vi "RT fast measure v2.vi"(8 "error in":errorcluster, 11 "FPGA DAQ1":refnum<k20>) -> (0 "error out":errorcluster)   [LabVIEW 2024]
uses:
  RT fast data.ctl
  <vilib>/LabVIEW Targets/FPGA/cRIO/shared/nicrio_ModuleControls/nicrio_cRIO-9775_RecordDataRates4ChansRing.ctl
  <vilib>/LabVIEW Targets/FPGA/cRIO/shared/nicrio_ModuleControls/nicrio_BasicConversionTime.ctl
  Ramps.ctl
  <vilib>/FPGAPlugInAG/Dynamic/niLvFpga_Reset_Dynamic.vi
  <vilib>/Utility/error.llb/Error Cluster From Error Code.vi
  <vilib>/rvi/errors/niLvFpgaAdjustHostInterfaceError.vi
  <vilib>/FPGAPlugInAG/Dynamic/niLvFpga_Run_Dynamic.vi
  <vilib>/RVI Host/nirviSupport.llb/nirviErrorClusterFromErrorCode.vi
  <vilib>/rvi/interface/nirviMethod/nirviMethod.xnode
  <vilib>/rvi/interface/nirviReadWriteControl/nirviReadWriteControl.xnode
  <resource>/objmgr/ni.dex.rc
  <vilib>/rvi/interface/nirviMethod/StockFPGA_InlinedMethodWaitForSingleIRQ.vi
  <vilib>/FPGAPlugInAG/Dynamic/niLvFpga_WaitOnIrq_Dynamic.vi
  <vilib>/FPGAPlugInAG/Dynamic/niLvFpga_AcknowledgeIrq_Dynamic.vi
  <vilib>/FPGAPlugInAG/Dynamic/niLvFpga_ReadFifo_Dynamic.vi
  <vilib>/rvi/errors/niLvFpgaMergeErrorWithErrorCode.vi
  NiFpgaLv.dll
  <vilib>/rvi/interface/Simulation/niFpgaSimulationCallBeginRW.vi
panel:
  in  "Parameters":T1={"Records Num"=10000, "AI Trigger Configuration"={"Trigger Slope"=enum."Positive", "Trigger Level"=0.1298828125, "Hystesis Value"=0.0, "AI Channel"=0}, "Record PreTrigger Samples"=1, "Record Samples"=16, "Ic Cut off or curve"=TRUE, "Record Data Rate"=1, "Wait before trigger us"=10100, "Cutoff delay usec"=0, "Timing Mode"=enum."High Resolution", "Trigger length ticks"=15000, "Timeout"=-1, "Ramps"={"Amp"=0.0, "Delay time 10us"=1, "Ramp1 time 10us"=1000, "Ramp2 time 10us"=2000, "Ramp3 time 10us"=1000, "End time 10us"=1}} {"Record Data Rate" items=["20.000 MS/s (NI 9775)"=1, "10.00 MS/s (NI 9775)"=2, "6.667 MS/s (NI 9775)"=3, "5.000 MS/s (NI 9775)"=4, "2.500 MS/s (NI 9775)"=8, "1.667 MS/s (NI 9775)"=12, "1.250 MS/s (NI 9775)"=16, "1.000 MS/s (NI 9775)"=20, "833.333 KS/s (NI 9775)"=24, "714.286 KS/s (NI 9775)"=28, "625.000 KS/s (NI 9775)"=32, "555.556 KS/s (NI 9775)"=36, "500.000 KS/s (NI 9775)"=40, "454.545 KS/s (NI 9775)"=44, "416.667 KS/s (NI 9775)"=48, "384.615 KS/s (NI 9775)"=52, "357.143 KS/s (NI 9775)"=56, "333.333 KS/s (NI 9775)"=60, "312.500 KS/s (NI 9775)"=64, "294.118 KS/s (NI 9775)"=68, "277.778 KS/s (NI 9775)"=72, "263.158 KS/s (NI 9775)"=76, "250.000 KS/s (NI 9775)"=80, "238.095 KS/s (NI 9775)"=84, "227.273 KS/s (NI 9775)"=88, "217.391 KS/s (NI 9775)"=92, "208.333 KS/s (NI 9775)"=96, "200.000 KS/s (NI 9775)"=100, "192.308 KS/s (NI 9775)"=104, "185.185 KS/s (NI 9775)"=108, "178.571 KS/s (NI 9775)"=112, "172.414 KS/s (NI 9775)"=116, "166.667 KS/s (NI 9775)"=120, "161.290 KS/s (NI 9775)"=124, "156.250 KS/s (NI 9775)"=128, "151.515 KS/s (NI 9775)"=132, "147.059 KS/s (NI 9775)"=136, "142.857 KS/s (NI 9775)"=140, "138.889 KS/s (NI 9775)"=144, "135.135 KS/s (NI 9775)"=148, "131.579 KS/s (NI 9775)"=152, "128.205 KS/s (NI 9775)"=156, "125.000 KS/s (NI 9775)"=160, "121.951 KS/s (NI 9775)"=164, "119.048 KS/s (NI 9775)"=168, "116.279 KS/s (NI 9775)"=172, "113.636 KS/s (NI 9775)"=176, "111.111 KS/s (NI 9775)"=180, "108.696 KS/s (NI 9775)"=184, "106.383 KS/s (NI 9775)"=188, "104.167 KS/s (NI 9775)"=192, "102.041 KS/s (NI 9775)"=196, "100.000 KS/s (NI 9775)"=200, "50.000 KS/s (NI 9775)"=400, "33.333 KS/s (NI 9775)"=600, "25.000 KS/s (NI 9775)"=800, "20.000 KS/s (NI 9775)"=1000, "16.667 KS/s (NI 9775)"=1200, "14.286 KS/s (NI 9775)"=1400, "12.500 KS/s (NI 9775)"=1600, "11.111 KS/s (NI 9775)"=1800, "10.000 KS/s (NI 9775)"=2000, "9.091 KS/s (NI 9775)"=2200, "8.333 KS/s (NI 9775)"=2400, "7.692 KS/s (NI 9775)"=2600, "7.143 KS/s (NI 9775)"=2800, "6.667 KS/s (NI 9775)"=3000, "6.250 KS/s (NI 9775)"=3200, "5.882 KS/s (NI 9775)"=3400, "5.556 KS/s (NI 9775)"=3600, "5.000 KS/s (NI 9775)"=4000, "4.762 KS/s (NI 9775)"=4200, "4.545 KS/s (NI 9775)"=4400, "4.348 KS/s (NI 9775)"=4600, "4.167 KS/s (NI 9775)"=4800, "4.000 KS/s (NI 9775)"=5000, "3.846 KS/s (NI 9775)"=5200, "3.571 KS/s (NI 9775)"=5600, "3.333 KS/s (NI 9775)"=6000, "3.125 KS/s (NI 9775)"=6400, "2.941 KS/s (NI 9775)"=6800, "2.778 KS/s (NI 9775)"=7200, "2.632 KS/s (NI 9775)"=7600, "2.500 KS/s (NI 9775)"=8000, "2.381 KS/s (NI 9775)"=8400, "2.273 KS/s (NI 9775)"=8800, "2.174 KS/s (NI 9775)"=9200, "2.083 KS/s (NI 9775)"=9600, "2.000 KS/s (NI 9775)"=10000, "1.923 KS/s (NI 9775)"=10400, "1.852 KS/s (NI 9775)"=10800, "1.786 KS/s (NI 9775)"=11200, "1.724 KS/s (NI 9775)"=11600, "1.667 KS/s (NI 9775)"=12000, "1.613 KS/s (NI 9775)"=12400, "1.563 KS/s (NI 9775)"=12800, "1.515 KS/s (NI 9775)"=13200, "1.471 KS/s (NI 9775)"=13600, "1.429 KS/s (NI 9775)"=14000, "1.389 KS/s (NI 9775)"=14400, "1.351 KS/s (NI 9775)"=14800, "1.316 KS/s (NI 9775)"=15200, "1.282 KS/s (NI 9775)"=15600, "1.250 KS/s (NI 9775)"=16000, "1.220 KS/s (NI 9775)"=16400, "1.190 KS/s (NI 9775)"=16800, "1.163 KS/s (NI 9775)"=17200, "1.136 KS/s (NI 9775)"=17600, "1.111 KS/s (NI 9775)"=18000, "1.087 KS/s (NI 9775)"=18400, "1.064 KS/s (NI 9775)"=18800, "1.042 KS/s (NI 9775)"=19200, "1.020 KS/s (NI 9775)"=19600, "1.000 KS/s (NI 9775)"=20000, "0.980 KS/s (NI 9775)"=20400, "0.962 KS/s (NI 9775)"=20800, "0.943 KS/s (NI 9775)"=21200, "0.926 KS/s (NI 9775)"=21600, "0.909 KS/s (NI 9775)"=22000, "0.893 KS/s (NI 9775)"=22400, "0.877 KS/s (NI 9775)"=22800, "0.862 KS/s (NI 9775)"=23200, "0.847 KS/s (NI 9775)"=23600, "0.833 KS/s (NI 9775)"=24000, "0.820 KS/s (NI 9775)"=24400, "0.806 KS/s (NI 9775)"=24800, "0.794 KS/s (NI 9775)"=25200, "0.781 KS/s (NI 9775)"=25600, "0.694 KS/s (NI 9775)"=28800, "0.625 KS/s (NI 9775)"=32000, "0.568 KS/s (NI 9775)"=35200, "0.521 KS/s (NI 9775)"=38400, "0.446 KS/s (NI 9775)"=44800, "0.391 KS/s (NI 9775)"=51200, "0.347 KS/s (NI 9775)"=57600, "0.313 KS/s (NI 9775)"=64000]}
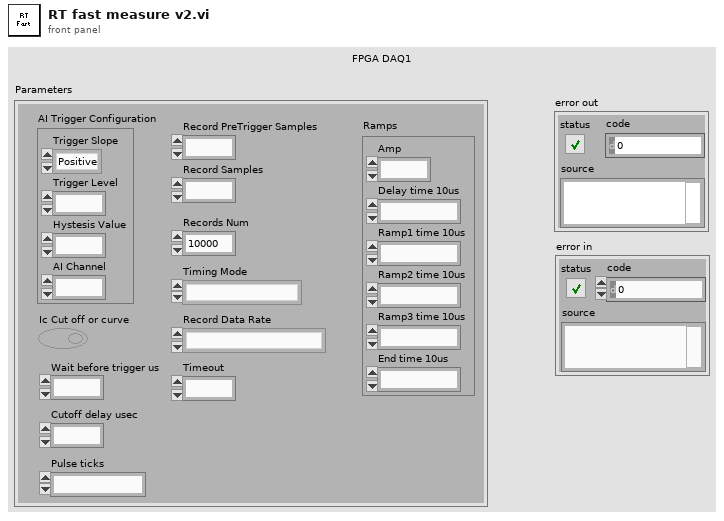
[diagram p1: front panel]
types:
  T1 = typedef "RT fast data.ctl" = cluster{"Records Num":i32, "AI Trigger Configuration":cluster{"Trigger Slope":enum8{"Positive", "Negative"}, "Trigger Level":fxp<+/-,17,5>, "Hystesis Value":fxp<+,16,4>, "AI Channel":u8}, "Record PreTrigger Samples":u32, "Record Samples":u32, "Ic Cut off or curve":bool, "Record Data Rate":T2, "Wait before trigger us":u32, "Cutoff delay usec":u32, "Timing Mode":T3, "Trigger length ticks":u32, "Timeout":i32, "Ramps":T4}
  T2 = typedef "nicrio_cRIO-9775_RecordDataRates4ChansRing.ctl" = u16
  T3 = typedef "nicrio_BasicConversionTime.ctl" = enum8{"High Speed", "High Resolution"}
  T4 = typedef "Ramps.ctl" = cluster{"Amp":fxp<+/-,20,5>, "Delay time 10us":i32, "Ramp1 time 10us":i32, "Ramp2 time 10us":i32, "Ramp3 time 10us":i32, "End time 10us":i32}
  T5 = cluster{"Trigger Slope":enum8{"Positive", "Negative"}, "Trigger Level":fxp<+/-,17,5>, "Hystesis Value":fxp<+,16,4>, "AI Channel":u8}
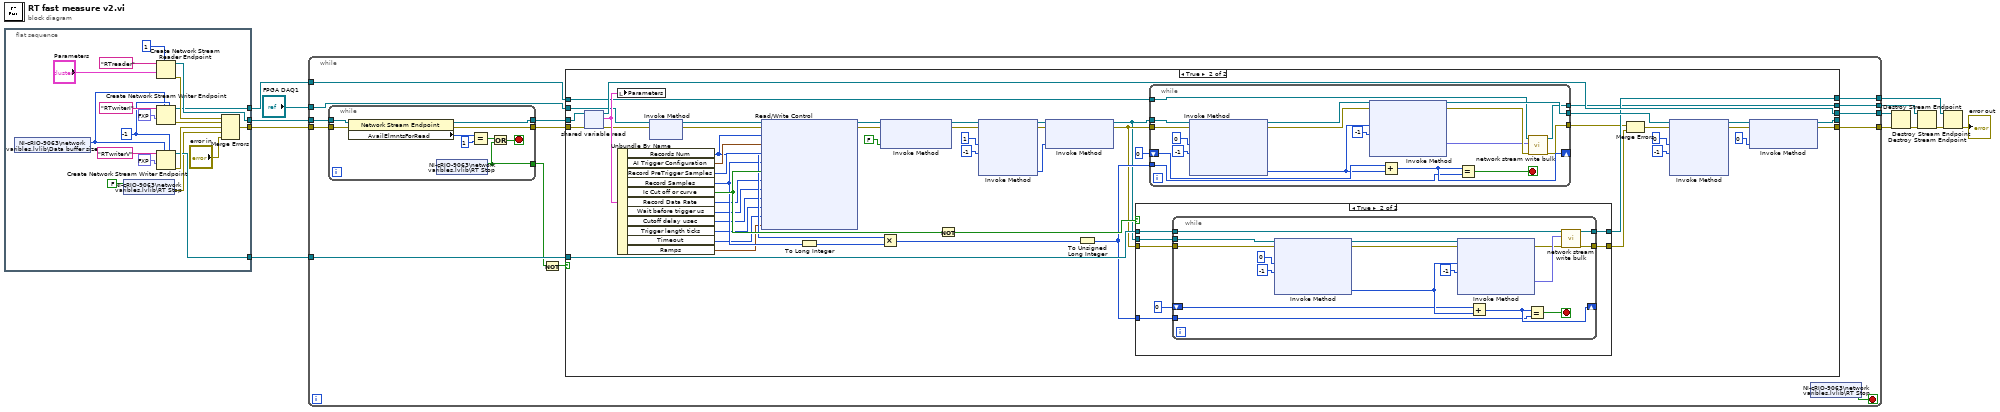
[diagram p0: block diagram]
diagram:
  n1 = flat-sequence {
    tunnel: [w29] -> w12
    tunnel: [w19] -> w11
    tunnel: [w18] -> w6
    tunnel: [w17] -> w5
    frame #0 {
      w24 = -1 ("timeout in ms (-1)")
      n2 = shared-variable "NI-cRIO-9063\\network varibles.lvlib\\Data buffer size"() -> (w23:i32)  [unwired: 1 in, 1 out]
      n3 = shared-variable "NI-cRIO-9063\\network varibles.lvlib\\RT Stop"(FALSE ("RT Stop")) -> (error out=w15:errorcluster)  [unwired: 1 in]
      n4 = Create Network Stream Reader Endpoint(7:1 ("reader buffer size"), 9:"Parameters", 11:"RTreader" ("reader name")) -> (0:w22:errorcluster, 3:w29:refnum<k21>)  [unwired: 4 in]
      n5 = Create Network Stream Writer Endpoint(5:w24, 7:w23, 9:fxp<+/-,17,5> 0.0, 11:"RTwriterI" ("writer name")) -> (0:w21:errorcluster, 3:w18:refnum<k21>)  [unwired: 3 in]
      n6 = Create Network Stream Writer Endpoint(5:w24, 7:w23, 9:fxp<+/-,17,5> 0.0, 11:"RTwriterV" ("writer name")) -> (0:w20:errorcluster, 3:w17:refnum<k21>)  [unwired: 3 in]
      n7 = Merge Errors(w22, w21, w20, w15, "error in") -> (w19:errorcluster)
    }
  }
  n8 = while {
    tunnel: w12 -> [w45]
    tunnel: w11 -> [w44]
    tunnel: [w34] -> w2
    tunnel: [w41] -> w10
    tunnel: w6 -> [w38]
    tunnel: w5 -> [w37]
    tunnel: [w36] -> w4
    tunnel: [w35] -> w3
    tunnel: "FPGA DAQ1" -> [w32]
    stop <- w40 stop-if-true
    n9 = while {
      tunnel: w45 -> [w154]
      tunnel: w44 -> [w153]
      tunnel: [w152] -> w43
      tunnel: [w151] -> w42
      tunnel: [w146] -> w33
      stop <- w147 stop-if-true
      n10 = property class="Network Stream Endpoint"(reference=w154, error in=w153) -> (reference out=w152:refnum<k21>, error out=w151:errorcluster, "AvailElmntsForRead"=w150:i32)
      n11 = shared-variable "NI-cRIO-9063\\network varibles.lvlib\\RT Stop"() -> (w146:bool)  [unwired: 1 in, 1 out]
      n12 = Equal?(x=w150, y=1) -> (x = y?=w148:bool)
      n13 = Or(x=w148, y=w146) -> (x .or. y?=w147:bool)
    }
    n14 = Not(x=w33) -> (.not. x?=w39:bool)
    n15 = case shown="True" w39 {
      tunnel: w43 -> [w49 w96]
      tunnel: w42 -> [w50 w65]
      tunnel: [w48 w88] -> _
      tunnel: [w50 w87] -> w34
      tunnel: [w49 w86] -> w41
      tunnel: w32 -> [w48 w66]
      tunnel: w38 -> [w47 w74]
      tunnel: w37 -> [w46 w76]
      tunnel: [w47 w73] -> w36
      tunnel: [w46 w75] -> w35
      frame False {
      }
      frame True {
        n16 = shared-variable-read(w96, w65) -> (w86:refnum<k21>, w64:errorcluster, w95:T1)  [unwired: 1 in, 1 out]
        n17 = local write "Parameters"(w95) -> ()
        n18 = Unbundle By Name(w95) -> ("Records Num"=w80:i32, "AI Trigger Configuration"=w98:T5, "Record PreTrigger Samples"=w97:u32, "Record Samples"=w79:u32, "Ic Cut off or curve"=w83:bool, "Record Data Rate"=w71:T2, "Wait before trigger us"=w67:u32, "Cutoff delay usec"=w63:u32, "Trigger length ticks"=w53:u32, "Timeout"=w52:i32, "Ramps"=w51:T4)
        n19 = xnode "Invoke Method"("FPGA VI Reference In"=w66, "error in"=w64) -> ("FPGA VI Reference Out"=w100:refnum<k20>, "error out"=w81:errorcluster)
        n20 = xnode "Read/Write Control"("FPGA VI Reference In"=w100, "error in"=w81, "Records Num"=w80, "AI Trigger Configuration"=w98, "Record PreTrigger Samples"=w97, "Record Samples"=w79, "Ic Cut off or curve"=w83, "Record Data Rate"=w71, "Wait before trigger us"=w67, "Cutoff delay usec"=w63, "Trigger length ticks"=w53, "Timeout"=w52, "Ramps"=w51) -> ("FPGA VI Reference Out"=w101:refnum<k20>, "error out"=w68:errorcluster)
        n21 = To Long Integer(number=w79) -> (32bit integer=w78:i32)
        n22 = xnode "Invoke Method"("FPGA VI Reference In"=w101, "error in"=w68, "Wait Until Done (F)"=FALSE) -> ("FPGA VI Reference Out"=w55:refnum<k20>, "error out"=w57:errorcluster)
        n23 = Multiply(x=w80, y=w78) -> (x*y=w77:i32)
        n24 = Not(x=w83) -> (.not. x?=w82:bool)
        n25 = xnode "Invoke Method"("FPGA VI Reference In"=w55, "error in"=w57, "IRQ Number(s)"=1, "Timeout (ms)"=-1) -> ("FPGA VI Reference Out"=w60:refnum<k20>, "error out"=w59:errorcluster, "IRQ(s) Asserted"=w58:i32)  [unwired: 1 out]
        n26 = xnode "Invoke Method"("FPGA VI Reference In"=w60, "error in"=w59, "IRQ Number(s)"=w58) -> ("FPGA VI Reference Out"=w54:refnum<k20>, "error out"=w56:errorcluster)
        n27 = To Unsigned Long Integer(number=w77) -> (unsigned 32bit integer=w69:u32)
        n28 = case shown="True" w82 {
          tunnel: w54 -> [_ w128]
          tunnel: [w120 w122] -> w85
          tunnel: w76 -> [w121 w127]
          tunnel: [w121 w123] -> w75
          tunnel: w56 -> [w120 w125]
          tunnel: w69 -> [_ w124]
          frame False {
          }
          frame True {
            n29 = while {
              tunnel: w128 -> [w138]
              tunnel: w127 -> [w133]
              shift-right: [w135] -> _
              shift-left: u32 0 ("Number of Elements") -> [w137]
              tunnel: w125 -> [w136]
              tunnel: w124 -> [w134]
              tunnel: [w132] -> w123
              tunnel: [w129] -> w122
              stop <- w139 stop-if-true
              n30 = xnode "Invoke Method"("FPGA VI Reference In"=w138, "error in"=w136, "Number of Elements"=u32 0, "Timeout (ms)"=-1) -> ("FPGA VI Reference Out"=w143:refnum<k20>, "error out"=w144:errorcluster, "Elements Remaining"=w145:u32)  [unwired: 1 out]
              n31 = xnode "Invoke Method"("FPGA VI Reference In"=w143, "error in"=w144, "Number of Elements"=w145, "Timeout (ms)"=-1) -> ("error out"=w130:errorcluster, "Data"=w131:fxp<+/-,17,5>[])  [unwired: 2 out]
              n32 = Add(x=w137, y=w145) -> (x+y=w135:u32)
              n33 = Equal?(x=w135, y=w134) -> (x = y?=w139:bool)
              n34 = call "network stream write bulk.vi"("error in (no error)"=w130, "Data"=w131, "endpoint in"=w133) -> ("error out"=w129:errorcluster, "endpoint out"=w132:refnum<k21>)  [unwired: 7 in]
            }
          }
        }
        n35 = while {
          tunnel: w74 -> [w103]
          tunnel: [w104] -> w73
          tunnel: w54 -> [w117]
          tunnel: [w118] -> w94
          tunnel: w56 -> [w115]
          tunnel: [w105] -> w72
          shift-right: [w109] -> _
          shift-left: u32 0 ("Number of Elements") -> [w111]
          tunnel: w69 -> [w108]
          stop <- w107 stop-if-true
          n36 = xnode "Invoke Method"("FPGA VI Reference In"=w117, "error in"=w115, "Number of Elements"=u32 0, "Timeout (ms)"=-1) -> ("FPGA VI Reference Out"=w116:refnum<k20>, "error out"=w114:errorcluster, "Elements Remaining"=w110:u32)  [unwired: 1 out]
          n37 = xnode "Invoke Method"("FPGA VI Reference In"=w116, "error in"=w114, "Number of Elements"=w110, "Timeout (ms)"=-1) -> ("FPGA VI Reference Out"=w118:refnum<k20>, "error out"=w106:errorcluster, "Data"=w102:fxp<+/-,17,5>[])  [unwired: 1 out]
          n38 = Add(x=w111, y=w110) -> (x+y=w109:u32)
          n39 = Equal?(x=w109, y=w108) -> (x = y?=w107:bool)
          n40 = call "network stream write bulk.vi"("error in (no error)"=w106, "Data"=w102, "endpoint in"=w103) -> ("error out"=w105:errorcluster, "endpoint out"=w104:refnum<k21>)  [unwired: 7 in]
        }
        n41 = Merge Errors(w72, w85) -> (w84:errorcluster)
        n42 = xnode "Invoke Method"("FPGA VI Reference In"=w94, "error in"=w84, "IRQ Number(s)"=0, "Timeout (ms)"=-1) -> ("FPGA VI Reference Out"=w91:refnum<k20>, "error out"=w90:errorcluster)  [unwired: 2 out]
        n43 = xnode "Invoke Method"("FPGA VI Reference In"=w91, "error in"=w90, "IRQ Number(s)"=0) -> ("FPGA VI Reference Out"=w88:refnum<k20>, "error out"=w87:errorcluster)
      }
    }
    n44 = shared-variable "NI-cRIO-9063\\network varibles.lvlib\\RT Stop"() -> (w40:bool)  [unwired: 1 in, 1 out]
  }
  n45 = Destroy Stream Endpoint(8:w2, 11:w10) -> (0:w9:errorcluster)
  n46 = Destroy Stream Endpoint(8:w9, 11:w4) -> (0:w8:errorcluster)
  n47 = Destroy Stream Endpoint(8:w8, 11:w3) -> (0:→"error out":errorcluster)
